vi "曲线属性.vi"(1 "大小":i32) -> (0 "曲线属性":T1[](array[typedef]))   [LabVIEW 2021]
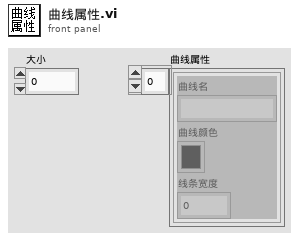
[diagram p1: front panel]
types:
  T1 = typedef "曲线属性.ctl" = cluster{"曲线名":string, "曲线颜色":u32, "线条宽度":u8}
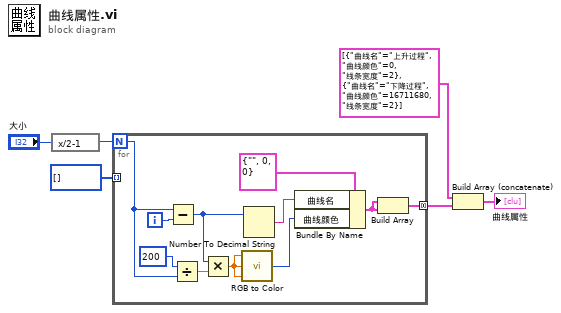
[diagram p0: block diagram]
diagram:
  n1 = expression code="x/2-1"("大小") -> (w6:i32)
  n2 = for {
    N: w6 -> [w16]
    tunnel: [w10] -> w4 mode=concatenating
    tunnel: i32[] [] ("添加的数组") -> [_] mode=indexing
    i -> [w15]
    n3 = Subtract(x=w16, y=w15) -> (x-y=w7:i32)
    n4 = Divide(x=200, y=w16) -> (x/y=w8:dbl)
    n5 = Multiply(x=w7, y=w8) -> (x*y=w14:dbl)
    n6 = call <vilib>:"RGB to Color.vi"("B"=w14, "G"=w14, "R"=w14) -> ("Color"=w12:u32)
    n7 = Number To Decimal String(number=w7) -> (decimal integer string=w9:string)  [unwired: 1 in]
    n8 = Bundle By Name(cluster=T1 {"曲线名"="", "曲线颜色"=0, "线条宽度"=0} ("曲线属性"), "曲线名"=w9, "曲线颜色"=w12) -> (w11:T1)
    n9 = Build Array(w11, w11) -> (w10:T1[])
  }
  n10 = Build Array (concatenate)(T1[] [{"曲线名"="上升过程", "曲线颜色"=0, "线条宽度"=2}, {"曲线名"="下降过程", "曲线颜色"=16711680, "线条宽度"=2}], w4) -> (→"曲线属性":T1[])
